vi "Rec Fetch Recordset Data (CR).vi"(4 "error in (no error)":errorcluster, 7 "command-recordset reference":T1) -> (0 "error out":errorcluster, 1 "recordset data":variant[][](array[variant]), 3 "command-recordset reference out":T1)   [LabVIEW 2013, in "NI_Database_API_64.lvlib"]
doc: "Retrieves the data in the recordset identified by the <B>recordset reference</B> input. You can convert each element in the array to its native LabVIEW data type using the Database Variant To Data function. Wire data to the reference input to determine the polymorphic instance to use or manually select the instance."
uses:
  NI_Database_API_64.lvlib
  Command-Recordset.llb/Cmd-Rec Object Reference.ctl
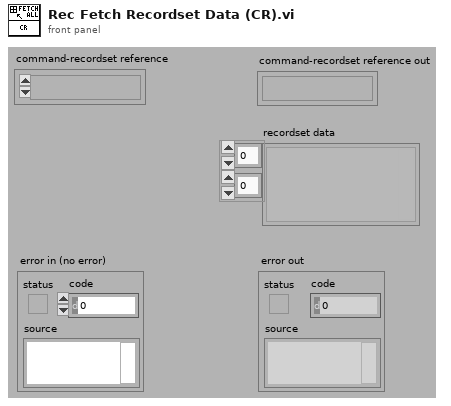
[diagram p1: front panel]
types:
  T1 = typedef "NI_Database_API_64.lvlib/Cmd-Rec Object Reference.ctl" = refnum<k1>
  T2 = typedef "NI_Database_API_64.lvlib/Cmd-Rec Data Members.ctl" = cluster{"recordset reference":T3, "command reference":T4}
  T3 = typedef "NI_Database_API_64.lvlib/Rec ObjectReference.ctl" = refnum<k1>
  T4 = typedef "NI_Database_API_64.lvlib/Cmd ObjectReference.ctl" = refnum<k1>
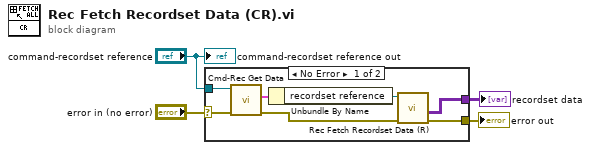
[diagram p0: block diagram]
diagram:
  n1 = case shown="No Error" "error in (no error)" {
    selector: "error in (no error)" -> [w6 w12]
    tunnel: [w11 w12] -> w4
    tunnel: [w9 _] -> w3
    tunnel: "command-recordset reference" -> [w7 _]
    frame No Error {
      n2 = call "Cmd-Rec Get Data.vi"("error in (no error)"=w6, "command-recordset reference"=w7) -> ("error out"=w5:errorcluster, "data"=w8:T2)  [unwired: 2 in, 2 out]
      n3 = Unbundle By Name(w8) -> ("recordset reference"=w10:T3)
      n4 = call "Rec Fetch Recordset Data (R).vi"("error in (no error)"=w5, "recordset reference"=w10) -> ("error out"=w11:errorcluster, "recordset data"=w9:variant[][])  [unwired: 3 in, 1 out]
    }
    frame Error {
    }
  }
  "error out" <- w4
  "recordset data" <- w3
  "command-recordset reference out" <- "command-recordset reference"
